vi "Galil_addresses_connection.vi"() -> ()   [LabVIEW 2011]
panel:
  in  "Galil.IGalil":refnum<k7>
  out "error out 2":errorcluster
  out "connection":string[](array[string])
  out "addresses":string[](array[string])
  out "Library Version:":string
  out "error out":errorcluster
  # "This vi Shows how to use the addresses member of the Galil Communications Library.  \n\nThis will list all of the available controllers on the PC/network"
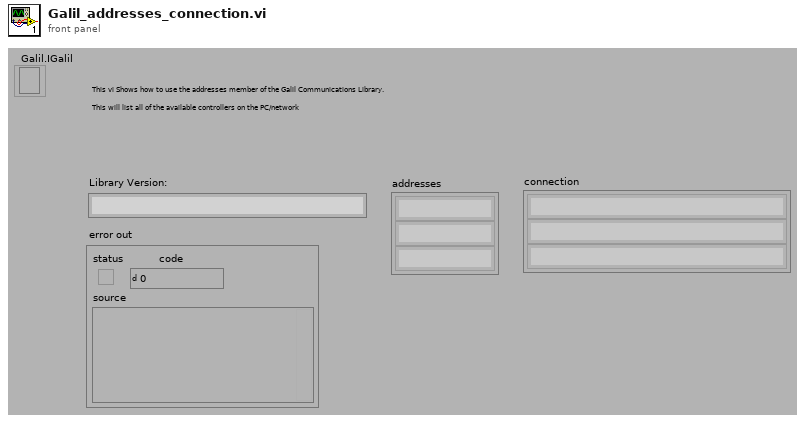
[diagram p1: front panel]
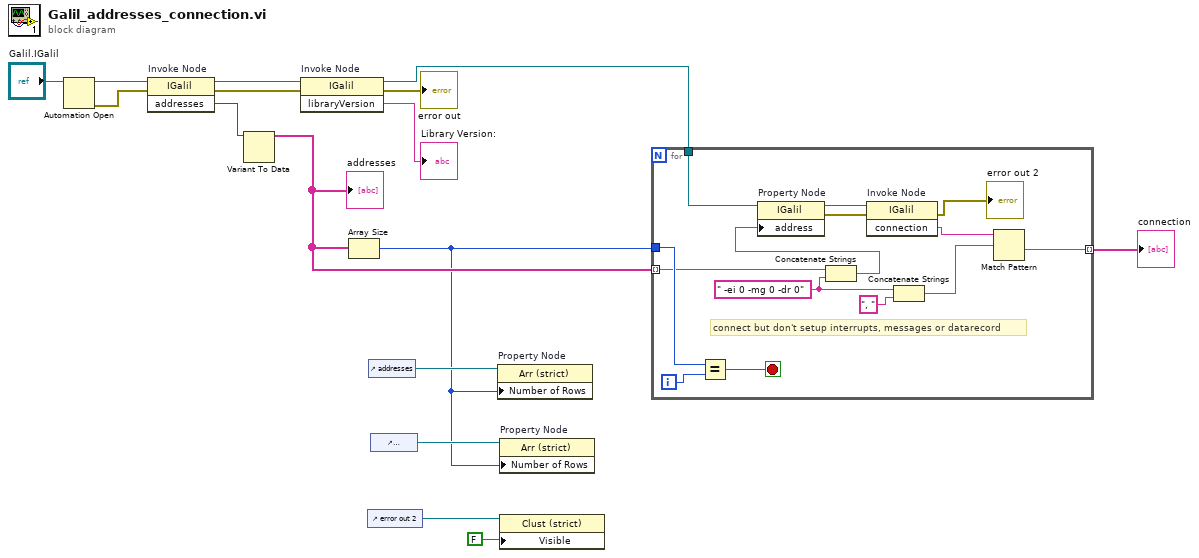
[diagram p0: block diagram]
diagram:
  n1 = Automation Open(Automation Refnum="Galil.IGalil") -> (Automation Refnum=w14:refnum<k7>, error out=w13:errorcluster)  [unwired: 1 in, 2 out]
  n2 = invoke on="Invoke Node" class="IGalil" method="addresses"(reference=w14, error in=w13) -> (reference out=w16:refnum<k7>, error out=w12:errorcluster, "addresses"=w11:variant)  [unwired: 1 in]
  n3 = Variant To Data(Variant=w11) -> (data=w8:string[])  [unwired: 2 in, 1 out]
  "addresses" <- w8
  n4 = invoke on="Invoke Node" class="IGalil" method="libraryVersion"(reference=w16, error in=w12) -> (reference out=w6:refnum<k7>, error out=→"error out":errorcluster, "libraryVersion"=→"Library Version:":string)  [unwired: 1 in]
  n5 = Array Size(array=w8) -> (size(s)=w4:i32)
  n6 = control-ref of="error out 2"() -> (w3:refnum<vi>)
  n7 = control-ref of="addresses"() -> (w9:refnum<vi>)
  n8 = control-ref of="connection"() -> (w5:refnum<vi>)
  n9 = property on="Property Node" class="Arr (strict)"(reference=w9, "Number of Rows"=w4) -> ()  [unwired: 1 in, 2 out]
  n10 = property on="Property Node" class="Arr (strict)"(reference=w5, "Number of Rows"=w4) -> ()  [unwired: 1 in, 2 out]
  n11 = property class="Clust (strict)"(reference=w3, "Visible"=FALSE) -> ()  [unwired: 1 in, 2 out]
  n12 = for {
    tunnel: w8 -> [w23] mode=indexing
    tunnel: [w20] -> w7 mode=indexing
    tunnel: w6 -> [w28]
    tunnel: w4 -> [w24]
    i -> [w30]
    stop <- w29 stop-if-true
    w19 = " -ei 0 -mg 0 -dr 0" ("string")
    # "connect but don't setup interrupts, messages or datarecord"
    n13 = Equal?(x=w24, y=w30) -> (x = y?=w29:bool)
    n14 = Concatenate Strings(w23, w19) -> (w22:string)
    n15 = property on="Property Node" class="IGalil"(reference=w28, "address"=w22) -> (reference out=w27:refnum<k7>, error out=w26:errorcluster)  [unwired: 1 in]
    n16 = invoke on="Invoke Node" class="IGalil" method="connection"(reference=w27, error in=w26) -> (error out=→"error out 2":errorcluster, "connection"=w21:string)  [unwired: 1 in, 1 out]
    n17 = Concatenate Strings(w19, ", " ("string")) -> (w17:string)
    n18 = Match Pattern(string=w21, regular expression=w17) -> (after substring=w20:string)  [unwired: 4 out]
  }
  "connection" <- w7
